vi "Create Upstream View SCM Spark Scene.vi"(2 "error in (no error)":errorcluster, 3 "Spark Coordinates (cm, rad, cm)":cluster{"r":sgl, "theta":sgl, "z":sgl}) -> (0 "error out":errorcluster, 1 "reference out":refnum<vi>)   [LabVIEW 2013, in "Breakdown Acoustics Controls.lvlib"]
uses:
  <vilib>/Utility/miscctls.llb/LV3DPointTypeDef.ctl
  <vilib>/picture/3D Picture Control/Object/Create Object (name).vi
  Breakdown Acoustics Controls.lvlib
  <vilib>/picture/3D Picture Control/NI_3D Picture Control.lvlib
panel:
  out "Cartesian\nCoordinates":cluster{"x":dbl, "y":dbl, "z":dbl}
  out "Spark Coordinates (cm, rad, rad)":cluster{"rho":dbl, "theta":dbl, "phi":dbl}
  out "Cavity Length (u)":sgl=1.2
  out "Cavity Radius (u)":sgl=1.2
  out "Graphical Units per Meter":dbl
  out "Cavity Upstream View":refnum<vi>(3d-picture)
  out "Spark Coordinates\n(cm, cm, cm)":T1
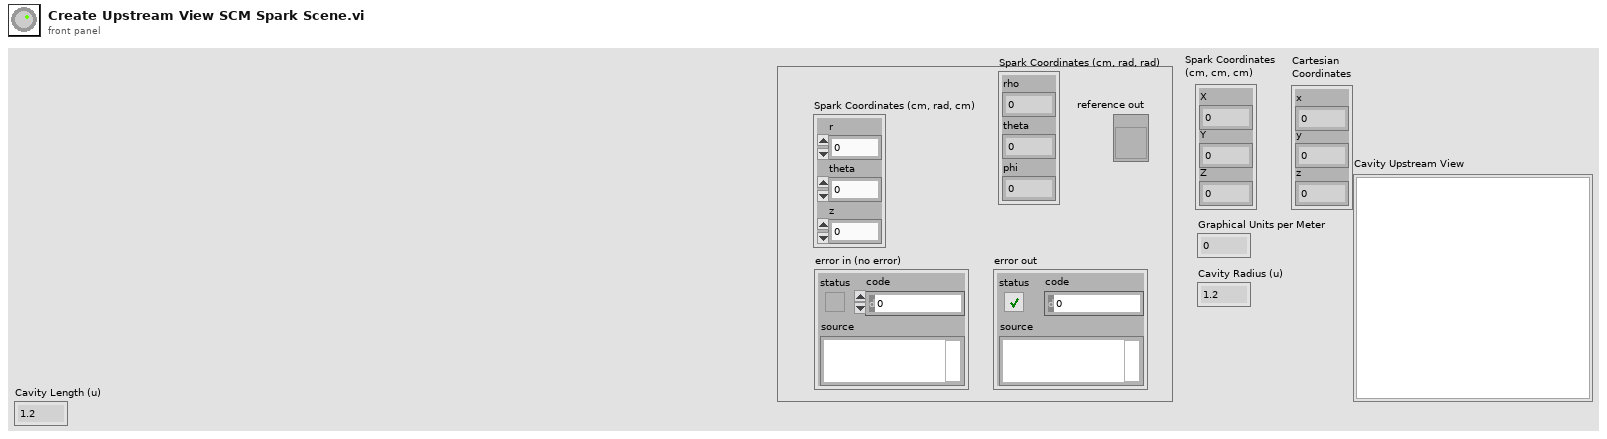
[diagram p1: front panel]
types:
  T1 = typedef "LV3DPointTypeDef.ctl" = cluster{"X":sgl, "Y":sgl, "Z":sgl}
  T2 = cluster{"Red":sgl, "Green":sgl, "Blue":sgl, "Alpha":sgl}
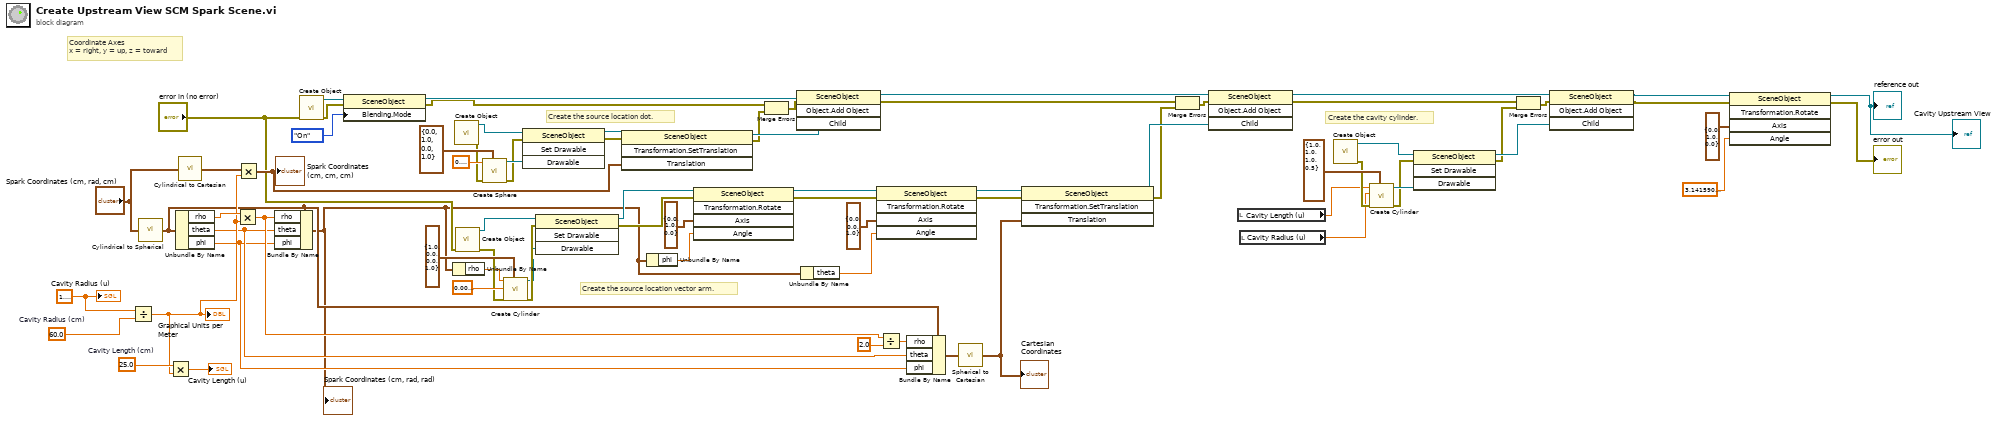
[diagram p0: block diagram]
diagram:
  w15 = sgl 25.0  # Cavity Length (cm)
  w61 = 60.0  # Cavity Radius (cm)
  w55 = sgl 1.2 ("Cavity Radius (u)")
  # "Coordinate Axes\nx = right, y = up, z = toward"
  # "Create the source location vector arm."
  # "Create the source location dot."
  # "Create the cavity cylinder."
  n1 = Divide ("graphical units per meter")(x=w55, y=w61) -> (x/y=w14:dbl)
  "Graphical Units per Meter" <- w14
  n2 = call "Cylindrical to Spherical.vi"("Cylindrical\nCoordinates"="Spark Coordinates (cm, rad, cm)") -> ("Spherical\nCoordinates"=w4:cluster{"rho":dbl, "theta":dbl, "phi":dbl})  [unwired: 4 in]
  n3 = Multiply(x=w15, y=w14) -> (x*y=→"Cavity Length (u)":dbl)
  n4 = Unbundle By Name(w4) -> ("rho"=w19:dbl, "theta"=w6:dbl, "phi"=w5:dbl)
  n5 = call "Cylindrical to Cartesian.vi"("Cylindrical\nCoordinates"="Spark Coordinates (cm, rad, cm)") -> ("Cartesian\nCoordinates"=w17:cluster{"x":dbl, "y":dbl, "z":dbl})  [unwired: 4 in]
  n6 = Multiply(x=w19, y=w14) -> (x*y=w7:dbl)
  n7 = Multiply(x=w17, y=w14) -> (x*y=w16:cluster{"x":dbl, "y":dbl, "z":dbl})
  "Spark Coordinates\n(cm, cm, cm)" <- w16
  n8 = Bundle By Name(cluster=w4, "rho"=w7, "theta"=w6, "phi"=w5) -> (w1:cluster{"rho":dbl, "theta":dbl, "phi":dbl})
  "Spark Coordinates (cm, rad, rad)" <- w1
  n9 = call-poly <vilib>:"Create Object.vi"("error in (no error)"="error in (no error)") -> ("error out"=w69:errorcluster, "Scene:New Object"=w70:refnum<vi>)  [unwired: 9 in]
  n10 = property class="SceneObject"(reference=w70, error in=w69, "Blending.Mode"=enum16{"Inherit Value", "Off", "On"}."On" ("Blending:Mode")) -> (reference out=w68:refnum<vi>, error out=w57:errorcluster)
  n11 = Unbundle By Name(w1) -> ("rho"=w18:dbl)
  n12 = call-poly <vilib>:"Create Object.vi"() -> ("error out"=w54:errorcluster, "Scene:New Object"=w66:refnum<vi>)  [unwired: 10 in]
  n13 = call-poly <vilib>:"Create Object.vi"("error in (no error)"="error in (no error)") -> ("error out"=w46:errorcluster, "Scene:New Object"=w48:refnum<vi>)  [unwired: 9 in]
  n14 = call <vilib>:"Create Sphere.vi"("Color"=T2 {"Red"=0.0, "Green"=1.0, "Blue"=0.0, "Alpha"=1.0}, "error in (no error)"=w54, "Radius"=sgl 0.1) -> ("error out"=w53:errorcluster, "New Sphere Refnum"=w72:refnum<vi>)  [unwired: 7 in]
  n15 = call <vilib>:"Create Cylinder.vi"("Color"=T2 {"Red"=1.0, "Green"=0.0, "Blue"=0.0, "Alpha"=1.0}, "error in (no error)"=w46, "Radius"=sgl 0.01, "Height"=w18) -> ("error out"=w45:errorcluster, "New Cylinder Refnum"=w37:refnum<vi>)  [unwired: 6 in]
  n16 = invoke class="SceneObject" method="Set Drawable"(reference=w66, error in=w53, "Drawable"=w72) -> (reference out=w64:refnum<vi>, error out=w63:errorcluster)  [unwired: 1 in, 2 out]
  n17 = invoke class="SceneObject" method="Set Drawable"(reference=w48, error in=w45, "Drawable"=w37) -> (reference out=w35:refnum<vi>, error out=w34:errorcluster)  [unwired: 1 in, 2 out]
  n18 = invoke class="SceneObject" method="Transformation.SetTranslation"(reference=w64, error in=w63, "Translation"=w16) -> (reference out=w60:refnum<vi>, error out=w58:errorcluster)  [unwired: 1 in, 2 out]
  n19 = Unbundle By Name(w1) -> ("phi"=w21:dbl)
  n20 = invoke class="SceneObject" method="Transformation.Rotate"(reference=w35, error in=w34, "Axis"=T1 {"X"=0.0, "Y"=1.0, "Z"=0.0}, "Angle"=w21) -> (reference out=w41:refnum<vi>, error out=w40:errorcluster)  [unwired: 1 in, 3 out]
  n21 = Merge Errors(w57, w58) -> (w59:errorcluster)
  n22 = invoke class="SceneObject" method="Object.Add Object"(reference=w68, error in=w59, "Child"=w60) -> (reference out=w32:refnum<vi>, error out=w31:errorcluster)  [unwired: 1 in, 2 out]
  n23 = Unbundle By Name(w1) -> ("theta"=w20:dbl)
  n24 = invoke class="SceneObject" method="Transformation.Rotate"(reference=w41, error in=w40, "Axis"=T1 {"X"=0.0, "Y"=0.0, "Z"=1.0}, "Angle"=w20) -> (reference out=w39:refnum<vi>, error out=w38:errorcluster)  [unwired: 1 in, 3 out]
  n25 = Divide(x=w7, y=2.0) -> (x/y=w9:dbl)
  n26 = Bundle By Name(cluster=w4, "rho"=w9, "theta"=w6, "phi"=w5) -> (w3:cluster{"rho":dbl, "theta":dbl, "phi":dbl})
  n27 = call "Spherical to Cartesian.vi"("Spherical\nCoordinates"=w3) -> ("Cartesian\nCoordinates"=w2:cluster{"x":dbl, "y":dbl, "z":dbl})  [unwired: 4 in]
  "Cartesian\nCoordinates" <- w2
  n28 = invoke class="SceneObject" method="Transformation.SetTranslation"(reference=w39, error in=w38, "Translation"=w2) -> (reference out=w36:refnum<vi>, error out=w33:errorcluster)  [unwired: 1 in, 2 out]
  n29 = Merge Errors(w31, w33) -> (w44:errorcluster)
  n30 = invoke class="SceneObject" method="Object.Add Object"(reference=w32, error in=w44, "Child"=w36) -> (reference out=w30:refnum<vi>, error out=w29:errorcluster)  [unwired: 1 in, 2 out]
  n31 = local read "Cavity Length (u)"() -> (w12:sgl)
  n32 = local read "Cavity Radius (u)"() -> (w11:sgl)
  n33 = call-poly <vilib>:"Create Object.vi"() -> ("error out"=w52:errorcluster, "Scene:New Object"=w65:refnum<vi>)  [unwired: 10 in]
  n34 = call <vilib>:"Create Cylinder.vi"("Color"=T2 {"Red"=1.0, "Green"=1.0, "Blue"=1.0, "Alpha"=0.5}, "error in (no error)"=w52, "Radius"=w11, "Height"=w12) -> ("error out"=w51:errorcluster, "New Cylinder Refnum"=w71:refnum<vi>)  [unwired: 6 in]
  n35 = invoke class="SceneObject" method="Set Drawable"(reference=w65, error in=w51, "Drawable"=w71) -> (reference out=w62:refnum<vi>, error out=w50:errorcluster)  [unwired: 1 in, 2 out]
  n36 = Merge Errors(w29, w50) -> (w56:errorcluster)
  n37 = invoke class="SceneObject" method="Object.Add Object"(reference=w30, error in=w56, "Child"=w62) -> (reference out=w24:refnum<vi>, error out=w23:errorcluster)  [unwired: 1 in, 2 out]
  n38 = invoke class="SceneObject" method="Transformation.Rotate"(reference=w24, error in=w23, "Axis"=T1 {"X"=0.0, "Y"=1.0, "Z"=0.0}, "Angle"=sgl 3.14159) -> (reference out=→"reference out" →"Cavity Upstream View":refnum<vi>, error out=→"error out":errorcluster)  [unwired: 1 in, 3 out]
  "Cavity Radius (u)" <- w55
